vi "Save AC png.vi"(6 "View":string, 8 "error in (no error)":errorcluster, 9 "DesignRequest":T1, 10 "reference":refnum<k24>, 11 "application":refnum<k24>) -> (0 "error out":errorcluster, 1 "DesignRequest out":T1, 2 "reference out":refnum<k24>, 3 "application out":refnum<k24>)   [LabVIEW 2011]
uses:
  Autodesk.AutoCAD.Interop
  Design Request.ctl
  Variable cluster.ctl
  Design Server.lvlib
panel:
  out "Command":string
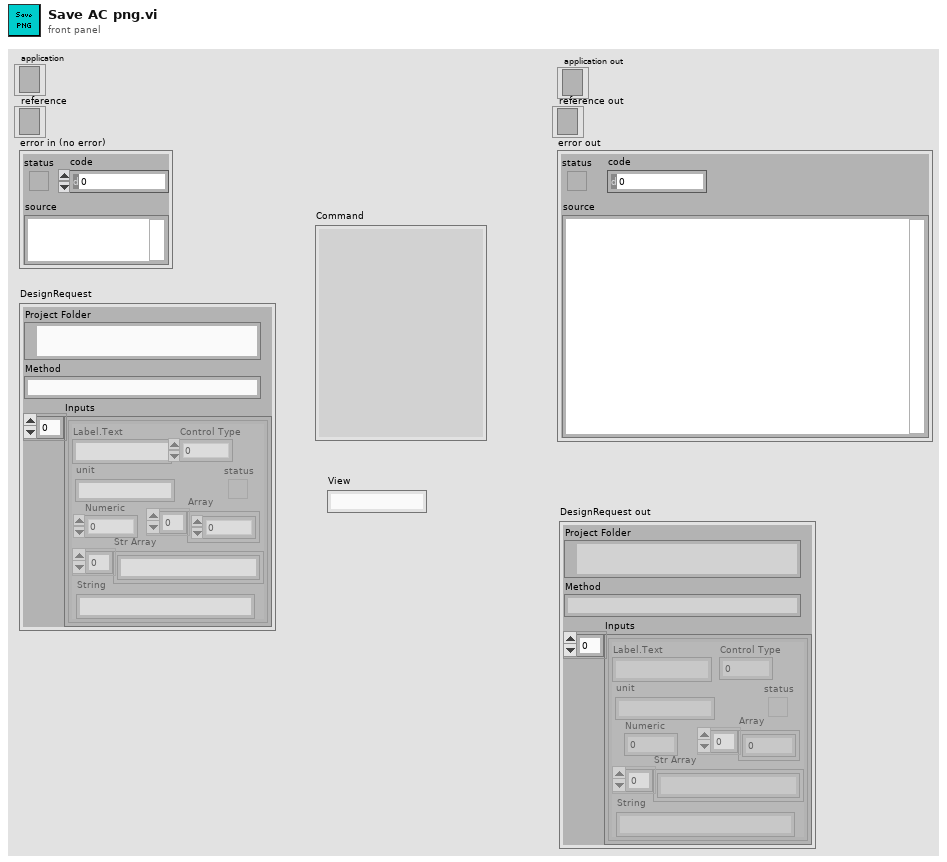
[diagram p1: front panel]
types:
  T1 = typedef "Design Server.lvlib/Design Request.ctl" = cluster{"Project Folder":path, "Method":string, "Inputs":T2}
  T2 = typedef "Design Server.lvlib/Variable cluster.ctl" = cluster{"Label.Text":string, "Control Type":u32, "Numeric":dbl, "Array":dbl[], "status":bool, "Str Array":string[], "String":string, "unit":string}[]
  T3 = typedef "imagedata.ctl" = cluster{"image type":i32, "image depth":i32, "image":u8[], "mask":u8[], "colors":u32[], "Rectangle":cluster{"left":i16, "top":i16, "right":i16, "bottom":i16}}
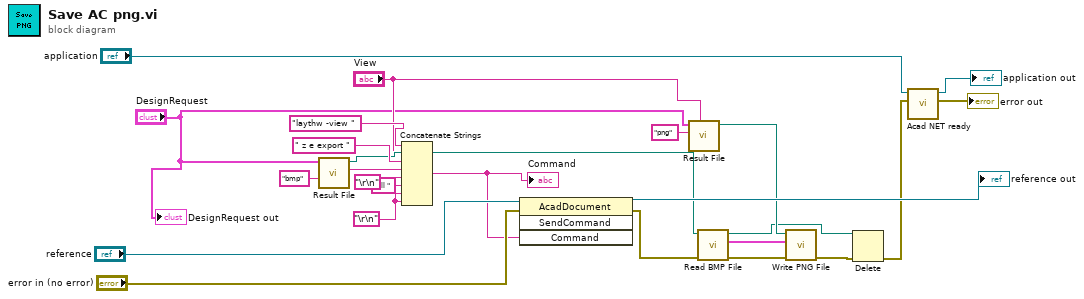
[diagram p0: block diagram]
diagram:
  w17 = "\r\n"
  n1 = call "Result File.vi"("File Type"="bmp", "DesignRequest"="DesignRequest") -> ("File string"=w14:string, "File path"=w13:path)  [unwired: 8 in]
  n2 = Concatenate Strings("laythw -view " ("string"), "View", " z e export " ("string"), w14, "\r\n", "all " ("string"), w17, w17) -> (w18:string)
  "Command" <- w18
  n3 = invoke class="AcadDocument" method="SendCommand"(reference="reference", error in="error in (no error)", "Command"=w18) -> (reference out=→"reference out":refnum<k24>, error out=w15:errorcluster)  [unwired: 1 in, 2 out]
  n4 = call "Result File.vi"("File name suffix"="View", "File Type"="png", "DesignRequest"="DesignRequest") -> ("File path"=w11:path)  [unwired: 7 in, 1 out]
  n5 = call <vilib>:"Read BMP File.vi"("error in (no error)"=w15, "path to BMP file"=w13) -> ("error out"=w16:errorcluster, "image data"=w1:T3, "path"=w9:path)  [unwired: 7 in]
  n6 = call <vilib>:"Write PNG File.vi"("error in (no error)"=w16, "image data"=w1, "path to PNG file"=w11) -> ("error out"=w10:errorcluster)  [unwired: 7 in, 1 out]
  n7 = Delete(path (use dialog)=w9, error in=w10) -> (error out=w6:errorcluster)  [unwired: 3 in, 2 out]
  n8 = call "Acad NET ready.vi"("error in (no error)"=w6, ".NET Refnum in"="application") -> ("error out"=→"error out":errorcluster, "reference out"=→"application out":refnum<k24>)  [unwired: 7 in, 1 out]
  "DesignRequest out" <- "DesignRequest"
